vi "Standard Engine.vi"(11 "engine references":T1) -> ()   [LabVIEW 2013, in "main engine.lvlib"]
doc: "This VI is a process that executes modules and has an API for transitioning through its state machine. Once it is initialized and running, it calls an array of module input methods, followed by an array of module process methods, followed by an array of module output methods, and then does any necessary error handling and bookkeeping."
uses:
  main engine.lvlib
  engine references.ctl
  <vilib>/NI/Module Execution Interface/Engine Runtime/Execution States.ctl
  Engine Data.ctl
  timed loop timing sources.ctl
  <vilib>/NI/Module Timing Source/timing source/TBM timing source.lvclass
  control loop data.ctl
  <vilib>/NI/Tag Bus/table/data table.ctl
  engine run schedule.ctl
  engine decimation schedule.ctl
  full module data.ctl
  <vilib>/NI/Tag Bus Module Framework/runtime/TBM module execution interface.lvclass
  module run state.ctl
  async executor/asynchronous executor reference.ctl
  async executor/message to executor.ctl
  Runtime/async command notification.ctl
  Runtime/async error info.ctl
  <vilib>/NI/Tag Bus Module Framework/runtime/error classification.ctl
  <vilib>/NI/Tag Bus Module Framework/module configuration/TBM module configuration.lvclass
  module method data.ctl
  <vilib>/NI/Tag Bus/table/transfer specification.ctl
  <vilib>/NI/Tag Bus/tag/Data Type.ctl
  fault handling spec.ctl
  Configuration/Error Actions.ctl
  status reporting data.ctl
  worker library/worker library reference.ctl
  worker library/worker comms.ctl
  worker library/worker commands.ctl
  worker library/request fifos.ctl
  worker library/recovery request.ctl
  worker library/rt fault.ctl
  worker library/response fifos.ctl
  worker library/recovery response.ctl
  <vilib>/NI/Module Execution Interface/Engine Runtime/Fault.ctl
  <vilib>/NI/Tag Bus/table/data table.lvlib
  <vilib>/NI/Tag Bus/tag/tag descriptor.lvclass
  Configuration/Standard Engine Configuration.lvclass
  async executor/async executor.lvlib
  <vilib>/NI/Module Execution Interface/Engine Runtime/Engine Runtime Interface.lvclass
  worker library/worker pool.lvlib
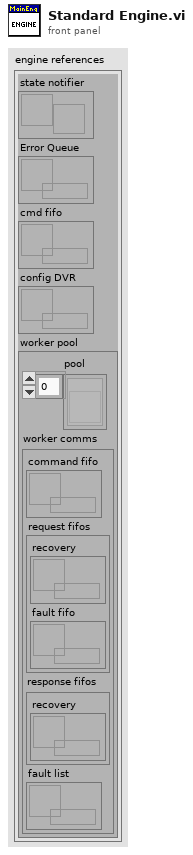
[diagram p1: front panel]
types:
  T1 = typedef "main engine.lvlib/engine references.ctl" = cluster{"state notifier":refnum<notifier>, "Error Queue":refnum<queue>, "cmd fifo":refnum<k33>, "config DVR":refnum<data-value>, "worker pool":T2}
  T2 = typedef "worker pool.lvlib/worker library reference.ctl" = cluster{"pool":refnum<vi>[], "worker comms":T3}
  T3 = typedef "worker pool.lvlib/worker comms.ctl" = cluster{"command fifo":refnum<k33>, "request fifos":T4, "response fifos":T5, "fault list":refnum<data-value>}
  T4 = typedef "worker pool.lvlib/request fifos.ctl" = cluster{"recovery":refnum<k33>, "fault fifo":refnum<k33>}
  T5 = typedef "worker pool.lvlib/response fifos.ctl" = cluster{"recovery":refnum<k33>}
  T6 = typedef "main engine.lvlib/Engine Data.ctl" = cluster{"timed loop timer source":T7, "control loop data":T8, "status reporting":T20}
  T7 = typedef "main engine.lvlib/timed loop timing sources.ctl" = cluster{"Processor":i32, "Priority":i32, "timing source dt":u32, "timer source":refnum<class "TBM timing source.lvclass">}
  T8 = typedef "main engine.lvlib/control loop data.ctl" = cluster{"engine tag bus":T9, "engine schedule":T10, "module information":T12[]}
  T9 = typedef "tag bus.lvlib/data table.lvlib/data table.ctl" = cluster{"Double":dbl[], "Single":sgl[], "I64":i64[], "I32":i32[], "I16":i16[], "I8":i8[], "U64":u64[], "U32":u32[], "U16":u16[], "U8":u8[], "Boolean":bool[], "String":string[], "Array of Double":cluster{"DBL Array":dbl[]}[], "Array of Single":cluster{"SGL Array":sgl[]}[], "Array of I64":cluster{"I64 Array":i64[]}[], "Array of I32":cluster{"I32 Array":i32[]}[], "Array of I16":cluster{"I16 Array":i16[]}[], "Array of I8":cluster{"I8 Array":i8[]}[], "Array of U64":cluster{"U64 Array":u64[]}[], "Array of U32":cluster{"U32 Array":u32[]}[], "Array of U16":cluster{"U16 Array":u16[]}[], "Array of U8":cluster{"U8 Array":u8[]}[], "Array of Boolean":cluster{"Boolean Array":bool[]}[], "Array of String":cluster{"String Array":string[]}[]}
  T10 = typedef "main engine.lvlib/engine run schedule.ctl" = cluster{"module run flags":u8[], "decimation schedule":T11}
  T11 = typedef "main engine.lvlib/engine decimation schedule.ctl" = cluster{"decimations":u16[], "offsets":u16[]}
  T12 = typedef "main engine.lvlib/full module data.ctl" = cluster{"run state":T13, "module":refnum<class "TBM module execution interface.lvclass">, "module ref":refnum<data-value>, "async exec ref":T14, "configuration ref":refnum<data-value>, "error":errorcluster, "previous error code":i32, "input method":T15, "output method":T15, "process method parameters":T15, "process method results":T15, "fault handling":T18, "error report index ":i32}
  T13 = typedef "main engine.lvlib/module run state.ctl" = enum16{"sync", "async"}
  T14 = typedef "async executor.lvlib/asynchronous executor reference.ctl" = cluster{"command fifo":refnum<k33>, "error fifo":refnum<k33>, "VI Refnum":refnum<vi>, "input buffer":refnum<k33>, "output buffer":refnum<k33>, "process buffer":refnum<k33>, "original dvrs":refnum<data-value>[]}
  T15 = typedef "main engine.lvlib/module method data.ctl" = cluster{"data table":T9, "transfer spec":T16[]}
  T16 = typedef "tag bus.lvlib/data table.lvlib/transfer specification.ctl" = cluster{"data type":T17, "sink indices":i32[], "source indices":i32[]}
  T17 = typedef "tag bus.lvlib/tag descriptor.lvclass/Data Type.ctl" = enum16{"Double", "Single", "I64", "I32", "I16", "I8", "U64", "U32", "U16", "U8", "Boolean", "String", "Array of Double", "Array of Single", "Array of I64", "Array of I32", "Array of I16", "Array of I8", "Array of U64", "Array of U32", "Array of U16", "Array of U8", "Array of Boolean", "Array of String"}
  T18 = typedef "main engine.lvlib/fault handling spec.ctl" = cluster{"unknown":T19[], "trivial":T19[], "critical":T19[], "recoverable":T19[]}
  T19 = typedef "Standard Engine Configuration.lvclass/Error Actions.ctl" = enum16{"Clear", "Notify", "Stop Component", "Stop Engine", "Safe State", "Attempt Recovery"}
  T20 = typedef "main engine.lvlib/status reporting data.ctl" = cluster{"late? index (bool)":i32, "late count index (U32)":i32, "dt (ns) index (U64)":i32}
  T21 = typedef "Engine Runtime Interface.lvclass/Execution States.ctl" = enum16{"Init", "Pre-Operational", "Safe-Operational", "Operational", "Stopped"}
  T22 = typedef "main engine.lvlib/engine process action.ctl" = enum16{"check for input", "load configuration", "unload configuration", "set safe outputs", "return to pre", "pre-run", "timed loop", "quit"}
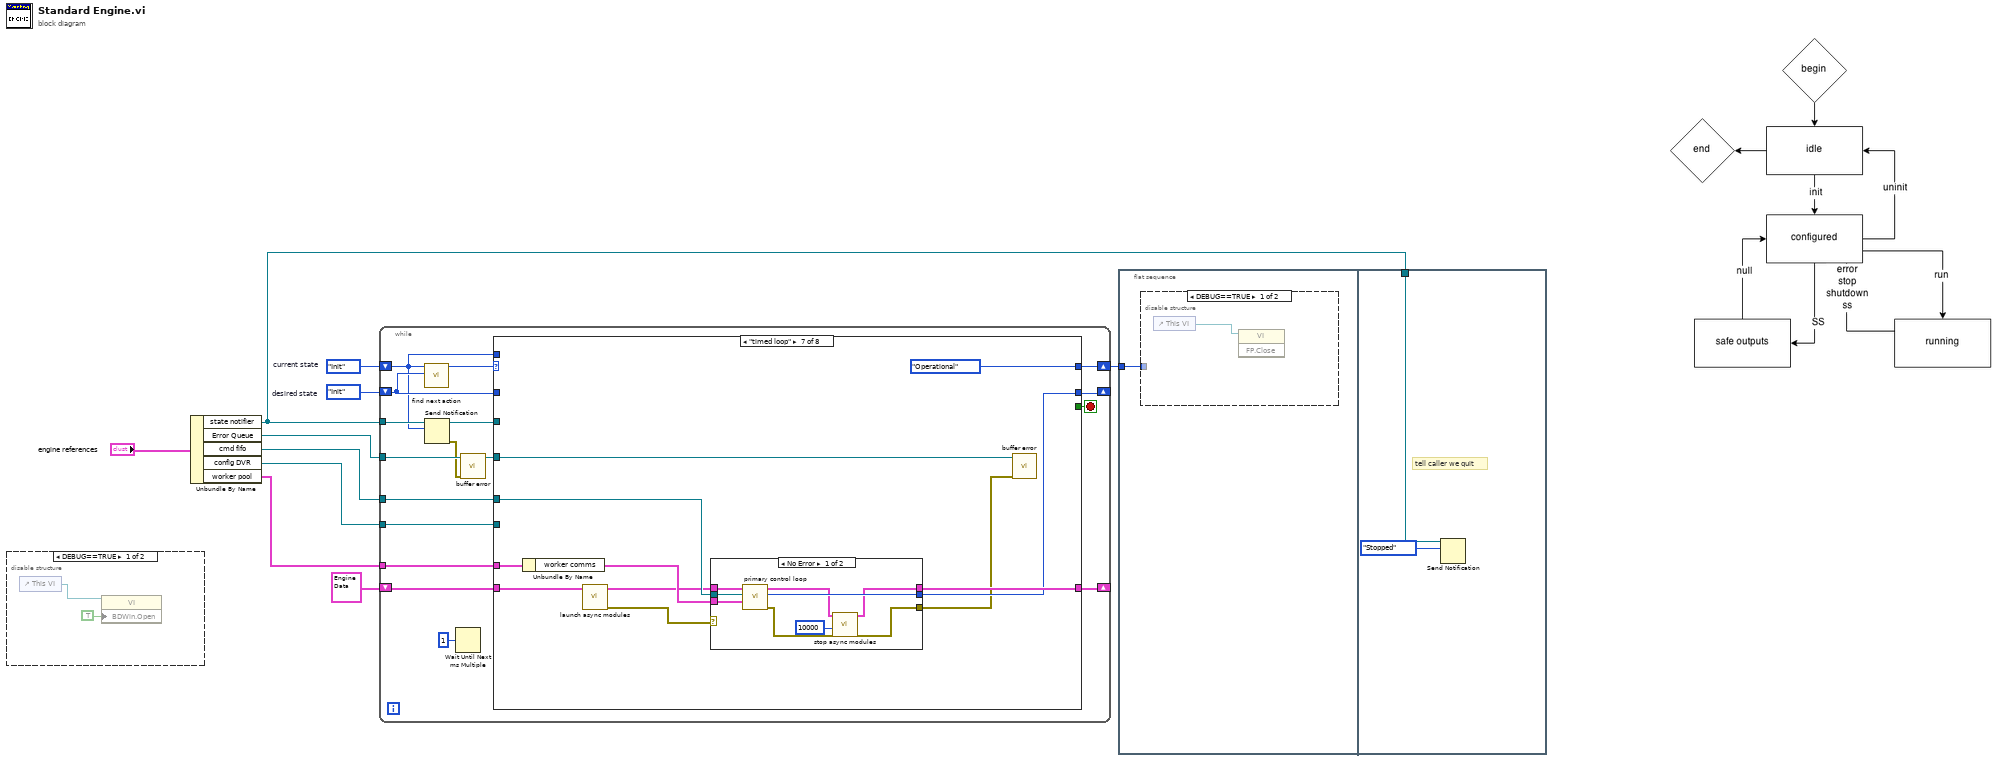
[diagram p0: block diagram]
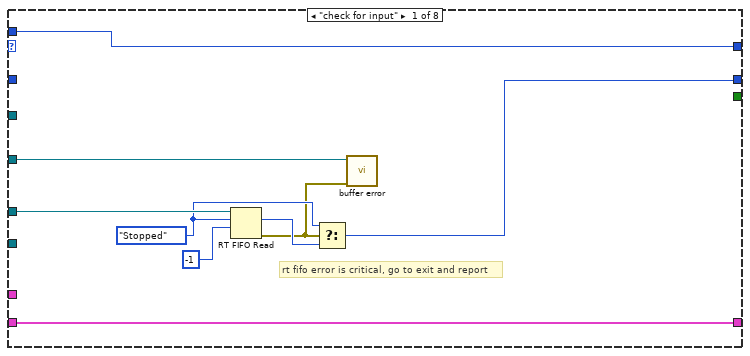
[diagram p4: hidden frame]
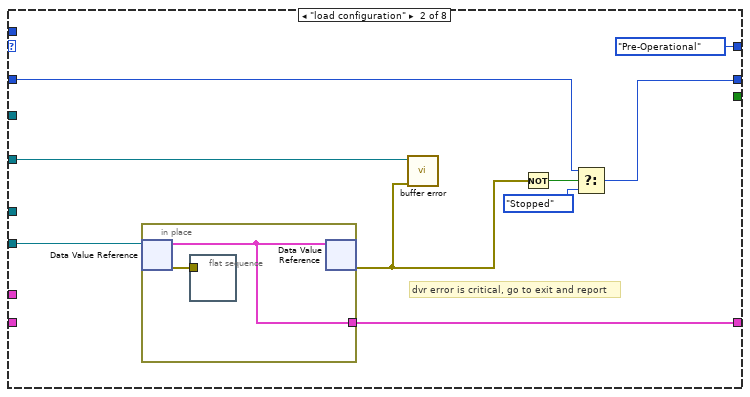
[diagram p5: hidden frame]
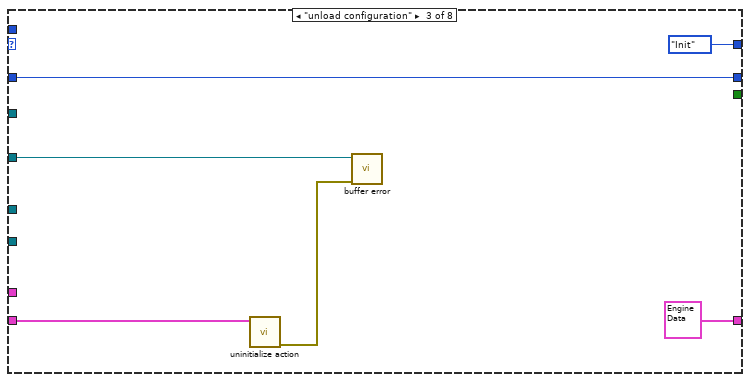
[diagram p6: hidden frame]
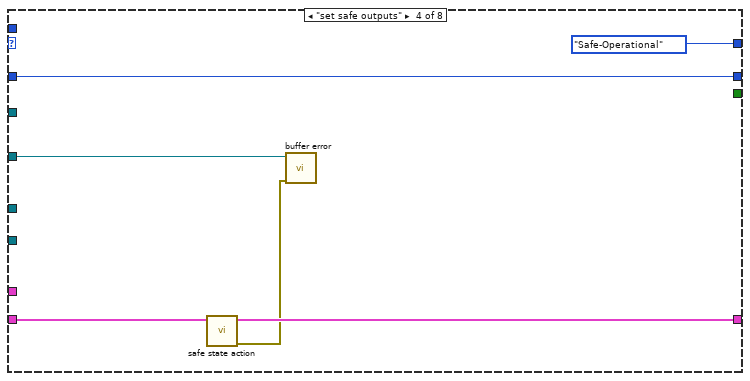
[diagram p7: hidden frame]
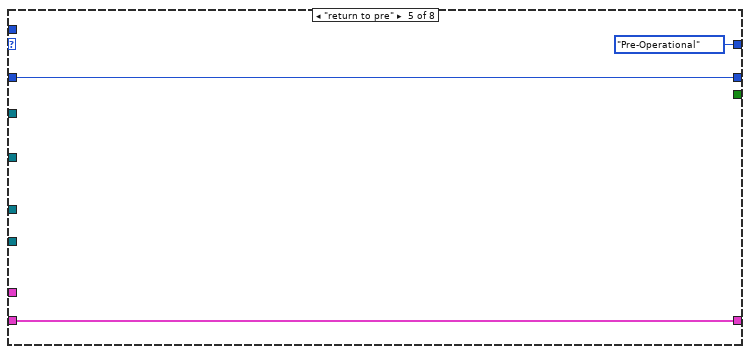
[diagram p8: hidden frame]
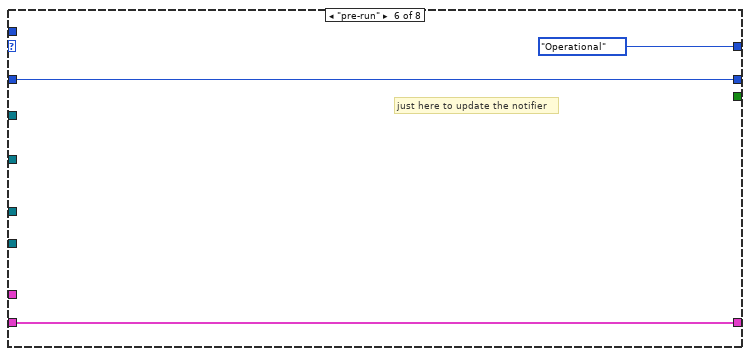
[diagram p9: hidden frame]
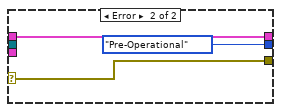
[diagram p10: hidden frame]
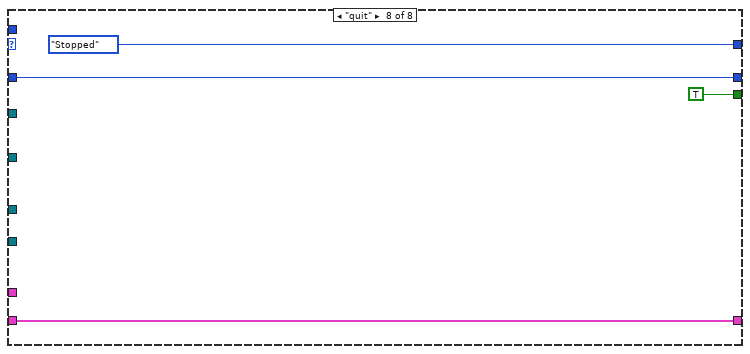
[diagram p11: hidden frame]
diagram:
  w9 = Execution_States."Init"  # desired state
  w10 = Execution_States."Init"  # current state
  n1 = disable-structure shown="DEBUG==TRUE" {
    frame condition #0 {
      n2 = control-ref of="This VI"() -> (w12:refnum<vi>)
      n3 = property class="VI"(reference=w12, "BDWin.Open"=TRUE ("Block Diagram Window:Open")) -> ()  [unwired: 1 in, 2 out]
    }
    frame condition #1 (active) {
    }
  }
  n4 = Unbundle By Name("engine references") -> ("state notifier"=w1:refnum<notifier>, "Error Queue"=w6:refnum<queue>, "cmd fifo"=w5:refnum<k33>, "config DVR"=w4:refnum<data-value>, "worker pool"=w3:T2)
  n5 = while {
    shift-right: [w27] -> w2
    shift-left: w10 -> [w23]
    shift-right: [w26] -> _
    shift-left: w9 -> [w28]
    tunnel: w1 -> [w24]
    tunnel: w6 -> [w22]
    tunnel: w5 -> [w19]
    tunnel: w4 -> [w18]
    shift-right: [w16] -> _
    shift-left: T6 {"timed loop timer source"={"Processor"=-2, "Priority"=0, "timing source dt"=0, "timer source"=refnum}, "control loop data"={"engine tag bus"={"Double"=[], "Single"=[], "I64"=[], "I32"=[], "I16"=[], "I8"=[], "U64"=[], "U32"=[], "U16"=[], "U8"=[], "Boolean"=[], "String"=[], "Array of Double"=[], "Array of Single"=[], "Array of I64"=[], "Array of I32"=[], "Array of I16"=[], "Array of I8"=[], "Array of U64"=[], "Array of U32"=[], "Array of U16"=[], "Array of U8"=[], "Array of Boolean"=[], "Array of String"=[]}, "engine schedule"={"module run flags"=[], "decimation schedule"={"decimations"=[], "offsets"=[]}}, "module information"=[]}, "status reporting"={"late? index (bool)"=0, "late count index (U32)"=0, "dt (ns) index (U64)"=0}} ("Engine Data Out") -> [w17]
    tunnel: w3 -> [w14]
    stop <- w25 stop-if-true
    n6 = call "find next action.vi"("desired state"=w28, "current state"=w23) -> ("action"=w29:T22)  [unwired: 9 in]
    n7 = Send Notification(notification=w23, notifier=w24) -> (notifier out=w13:refnum<notifier>, error out=w21:errorcluster)  [unwired: 1 in]
    n8 = Wait Until Next ms Multiple(millisecond multiple=u32 1) -> ()  [unwired: 1 out]
    n9 = call "buffer error.vi"("error in"=w21, "error buffer in"=w22) -> ("error buffer out"=w20:refnum<queue>)  [unwired: 9 in]
    n10 = case shown="\"timed loop\"" w29 {
      tunnel: w28 -> [_ w43 w55 w61 w64 w67 _ w94]
      tunnel: w23 -> [w38 _ _ _ _ _ _ _]
      tunnel: [w38 Execution_States."Pre-Operational" ("current state") Execution_States."Init" ("current state") Execution_States."Safe-Operational" ("current state") Execution_States."Pre-Operational" ("current state") Execution_States."Operational" ("current state") Execution_States."Operational" ("current state") Execution_States."Stopped" ("current state")] -> w27
      tunnel: [w33 w41 w55 w61 w64 w67 w74 w94] -> w26
      tunnel: [_ _ _ _ _ _ _ TRUE] -> w25
      tunnel: w20 -> [w32 w45 w52 w57 _ _ w75 _]
      tunnel: w19 -> [w37 _ _ _ _ _ w76 _]
      tunnel: w18 -> [_ w46 _ _ _ _ _ _]
      tunnel: w17 -> [w30 _ w53 w59 w63 w65 w69 w92]
      tunnel: [w30 w39 T6 {"timed loop timer source"={"Processor"=-2, "Priority"=0, "timing source dt"=0, "timer source"=refnum}, "control loop data"={"engine tag bus"={"Double"=[], "Single"=[], "I64"=[], "I32"=[], "I16"=[], "I8"=[], "U64"=[], "U32"=[], "U16"=[], "U8"=[], "Boolean"=[], "String"=[], "Array of Double"=[], "Array of Single"=[], "Array of I64"=[], "Array of I32"=[], "Array of I16"=[], "Array of I8"=[], "Array of U64"=[], "Array of U32"=[], "Array of U16"=[], "Array of U8"=[], "Array of Boolean"=[], "Array of String"=[]}, "engine schedule"={"module run flags"=[], "decimation schedule"={"decimations"=[], "offsets"=[]}}, "module information"=[]}, "status reporting"={"late? index (bool)"=0, "late count index (U32)"=0, "dt (ns) index (U64)"=0}} ("Engine Data Out") w58 w63 w65 w77 w92] -> w16
      tunnel: w14 -> [_ _ _ _ _ _ w72 _]
      tunnel: w13 -> [_ _ _ _ _ _ _ _]
      frame "check for input" {
        w35 = Execution_States."Stopped" ("element")
        # "rt fifo error is critical, go to exit and report"
        n11 = RT FIFO Read(0:w37, 1:w35, 2:-1 ("timeout in ms (0)")) -> (9:w34:T21, 11:w31:errorcluster)  [unwired: 1 in, 3 out]
        n12 = Select(t=w35, s=w31, f=w34) -> (s? t:f=w33:T21)
        n13 = call "buffer error.vi"("error in"=w31, "error buffer in"=w32) -> ()  [unwired: 9 in, 1 out]
      }
      frame "load configuration" {
        # "dvr error is critical, go to exit and report"
        n14 = in-place {
          in-place-border: [w49] -> w39
          n15 = in-place-dvr #1(w46) -> (w49:T6, w48:errorcluster)
          n16 = flat-sequence {
            tunnel: w48 -> [_]
            frame #0 {
            }
          }
          n17 = in-place-dvr #1(w49) -> (w44:errorcluster)  [unwired: 1 out]
        }
        n18 = call "buffer error.vi"("error in"=w44, "error buffer in"=w45) -> ()  [unwired: 9 in, 1 out]
        n19 = Not(x=w44) -> (.not. x?=w40:bool)
        n20 = Select(t=w43, s=w40, f=Execution_States."Stopped") -> (s? t:f=w41:T21)
      }
      frame "unload configuration" {
        n21 = call "uninitialize action.vi"("Engine Data Out in"=w53) -> ("error out"=w51:errorcluster)  [unwired: 10 in]
        n22 = call "buffer error.vi"("error in"=w51, "error buffer in"=w52) -> ()  [unwired: 9 in, 1 out]
      }
      frame "set safe outputs" {
        n23 = call "safe state action.vi"("Engine Data Out in"=w59) -> ("error out"=w56:errorcluster, "Engine Data Out out"=w58:T6)  [unwired: 9 in]
        n24 = call "buffer error.vi"("error in"=w56, "error buffer in"=w57) -> ()  [unwired: 9 in, 1 out]
      }
      frame "return to pre" {
      }
      frame "pre-run" {
        # "just here to update the notifier"
      }
      frame "timed loop" {
        n25 = Unbundle By Name(w72) -> ("worker comms"=w71:T3)
        n26 = call "launch async modules.vi"("Engine Data Out in"=w69) -> ("error out"=w68:errorcluster, "Engine Data Out out"=w70:T6)  [unwired: 9 in]
        n27 = case shown="No Error" w68 {
          selector: w68 -> [_ w88]
          tunnel: w70 -> [w87 w90]
          tunnel: [w83 w90] -> w77
          tunnel: w76 -> [w86 _]
          tunnel: [w85 Execution_States."Pre-Operational" ("desired state")] -> w74
          tunnel: [w81 w88] -> w73
          tunnel: w71 -> [w79 _]
          frame No Error {
            n28 = call "primary control loop.vi"("worker pool reference"=w79, "cmd fifo"=w86, "engine out"=w87) -> ("error out"=w82:errorcluster, "desired state"=w85:T21, "engine out"=w84:T6)  [unwired: 6 in]
            n29 = call "stop async modules.vi"("error in"=w82, "timeout (500 ms)"=u16 10000, "Engine Data Out in"=w84) -> ("error out"=w81:errorcluster, "Engine Data Out out"=w83:T6)  [unwired: 7 in]
          }
          frame Error {
          }
        }
        n30 = call "buffer error.vi"("error in"=w73, "error buffer in"=w75) -> ()  [unwired: 9 in, 1 out]
      }
      frame "quit" {
      }
    }
  }
  n31 = flat-sequence {
    tunnel: w2 -> [w95]
    tunnel: w1 -> [w97]
    frame #0 {
      n32 = disable-structure shown="DEBUG==TRUE" {
        disable-tunnel: w95 -> [_ _]
        frame condition #0 {
          n33 = control-ref of="This VI"() -> (w96:refnum<vi>)
          n34 = invoke class="VI" method="FP.Close"(reference=w96) -> ()  [unwired: 2 in, 3 out]
        }
        frame condition #1 (active) {
        }
      }
    }
    frame #1 {
      # "tell caller we quit"
      n35 = Send Notification(notification=Execution_States."Stopped" ("current state"), notifier=w97) -> ()  [unwired: 1 in, 2 out]
    }
  }
